vi "Execute.vi"(8 "error in (no error)":errorcluster, 9 "Consumer Queues in":T1, 10 "DAC Process Command in":refnum<class "Exit DAC.lvclass">, 11 "DAC Process Data in":T2) -> (0 "error out":errorcluster, 1 "Consumer Queues out":T1, 2 "Stop?":bool, 3 "DAC Process Data out":T2)   [LabVIEW 2019, in "DAC Process.lvlib" / "Exit DAC.lvclass"]
uses:
  Exit DAC.lvclass
  DAC Process Data.ctl
  Generic Test Stand/Generic Test Stand.lvclass
  TS Framework/ExeLogging/DAC Logger/DAC Logger.lvclass
  DAC State.ctl
  TS Framework/Consumer Queues.ctl
  UI Process/Generic UI Command/Generic UI Process Command.lvclass
  Generic DAC Command/Generic DAC Process Command.lvclass
  Trig Process/Generic Trig Command/Generic Trig Process Command.lvclass
  UI Process/Stop UI Process/Stop UI Process.lvclass
  Trig Process/Exit TRIG/Exit TRIG.lvclass
  Generic Test Stand/Generic Test Stand.lvclass/Generic Test Stand.ctl
  DAC Process.lvlib
  TS Framework/TS Framework.lvlib
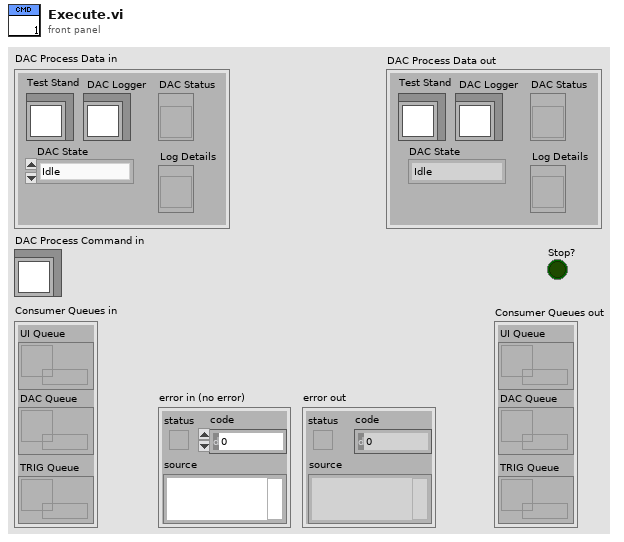
[diagram p1: front panel]
types:
  T1 = typedef "TS Framework.lvlib/Consumer Queues.ctl" = cluster{"UI Queue":refnum<queue>, "DAC Queue":refnum<queue>, "TRIG Queue":refnum<queue>}
  T2 = typedef "DAC Process.lvlib/DAC Process Data.ctl" = cluster{"Test Stand":refnum<class "Generic Test Stand.lvclass">, " DAC Logger":refnum<class "DAC Logger.lvclass">, "DAC State":T3, "DAC Status":refnum<vi>, "Log Details":refnum<vi>}
  T3 = typedef "DAC Process.lvlib/DAC State.ctl" = enum16{"Idle", "Acquiring"}
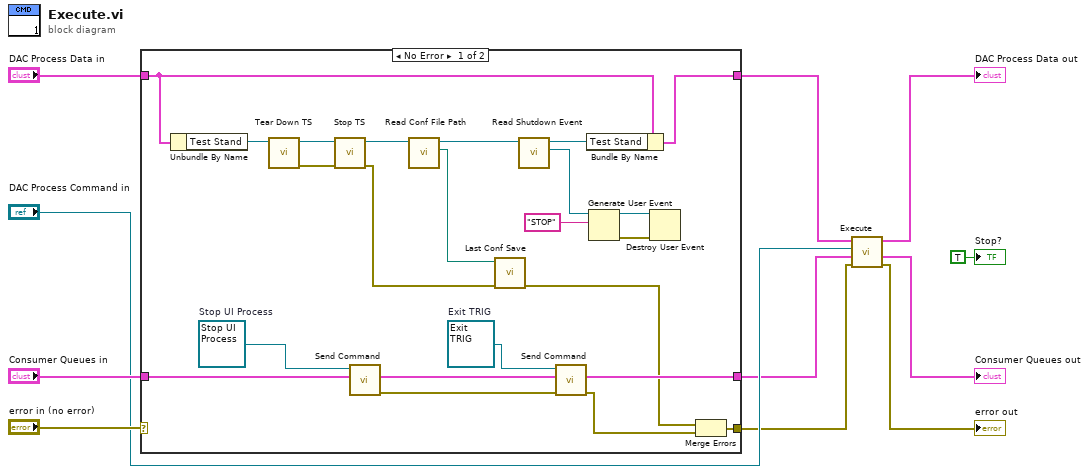
[diagram p0: block diagram]
diagram:
  n1 = case shown="No Error" "error in (no error)" {
    selector: "error in (no error)" -> [_ w37]
    tunnel: [w27 w37] -> w5
    tunnel: "DAC Process Data in" -> [w20 w36]
    tunnel: [w18 w36] -> w4
    tunnel: "Consumer Queues in" -> [w34 w35]
    tunnel: [w31 w35] -> w6
    frame No Error {
      w23 = refnum<class "Exit TRIG.lvclass"> refnum  # Exit TRIG
      w33 = refnum<class "Stop UI Process.lvclass"> refnum  # Stop UI Process
      n2 = Unbundle By Name(w20) -> ("Test Stand"=w22:refnum<class "Generic Test Stand.lvclass">)
      n3 = call-dynamic "Tear Down TS.vi"("Generic Test Stand in"=w22) -> ("error out"=w15:errorcluster, "Generic Test Stand out"=w17:refnum<class "Generic Test Stand.lvclass">)  [unwired: 9 in]
      n4 = call-dynamic "Stop TS.vi"("error in (no error)"=w15, "Generic Test Stand in"=w17) -> ("error out"=w14:errorcluster, "Generic Test Stand out"=w16:refnum<class "Generic Test Stand.lvclass">)  [unwired: 8 in]
      n5 = call-dynamic "Send Command.vi"("Consumer Queues in"=w34, "UI Process Command in"=w33) -> ("error out"=w25:errorcluster, "Consumer Queues out"=w32:T1)  [unwired: 8 in]
      n6 = call "Read Conf File Path.vi"("Generic Test Stand in"=w16) -> ("Conf File Path"=w24:path, "Generic Test Stand out"=w21:refnum<class "Generic Test Stand.lvclass">)  [unwired: 8 in, 1 out]
      n7 = call "Last Conf Save.vi"("error in"=w14, "Conf File"=w24) -> ("error out"=w13:errorcluster)  [unwired: 8 in]
      n8 = call "Read Shutdown Event.vi"("Generic Test Stand in"=w21) -> ("Shutdown Event"=w30:refnum<user-event>, "Generic Test Stand out"=w19:refnum<class "Generic Test Stand.lvclass">)  [unwired: 8 in, 1 out]
      n9 = call-dynamic "Send Command.vi"("error in (no error)"=w25, "Consumer Queues in"=w32, "Trig Process Command"=w23) -> ("error out"=w26:errorcluster, "Consumer Queues out"=w31:T1)  [unwired: 7 in]
      n10 = Bundle By Name(cluster=w20, "Test Stand"=w19) -> (w18:T2)
      n11 = Generate User Event(user event=w30, event data cluster="STOP" ("event data")) -> (user event out=w28:refnum<user-event>, error out=w12:errorcluster)  [unwired: 2 in]
      n12 = Destroy User Event(user event=w28, error in=w12) -> ()  [unwired: 1 out]
      n13 = Merge Errors(w13, w26) -> (w27:errorcluster)
    }
    frame Error {
    }
  }
  n14 = call-parent "Execute.vi"("error in"=w5, "Consumer Queues in"=w6, "DAC Process Command in"="DAC Process Command in", "DAC Process Data in"=w4) -> ("error out"=→"error out":errorcluster, "Consumer Queues out"=→"Consumer Queues out":T1, "DAC Process Data out"=→"DAC Process Data out":T2)  [unwired: 4 in, 1 out]
  "Stop?" <- TRUE ("Stop?")
